vi "DeleteDlls.vi"(11 "Destination Path":path) -> ()   [LabVIEW 2017]
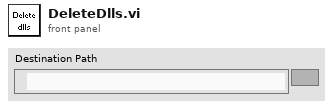
[diagram p1: front panel]
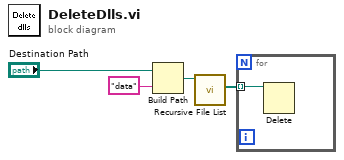
[diagram p0: block diagram]
diagram:
  n1 = Build Path(base path="Destination Path", name or relative path="data") -> (appended path=w2:path)
  n2 = call <vilib>:"Recursive File List.vi"("Folder Path"=w2) -> ("All Files in Dir"=w1:path[])  [unwired: 6 in, 4 out]
  n3 = for {
    tunnel: w1 -> [w5] mode=indexing
    n4 = Delete(path (use dialog)=w5) -> ()  [unwired: 4 in, 3 out]
  }
